vi "Quit LabVIEW.vi"(8 "error in (no error)":errorcluster) -> ()   [LabVIEW 2018]
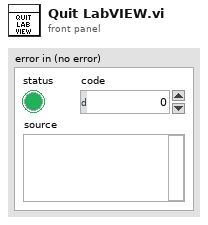
[diagram p1: front panel]
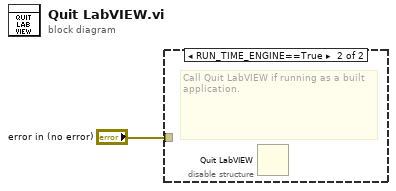
[diagram p0: block diagram]
diagram:
  n1 = disable-structure shown="RUN_TIME_ENGINE==True" {
    disable-tunnel: "error in (no error)" -> [_ _]
    frame condition #0 (active) {
    }
    frame condition #1 {
      # "Call Quit LabVIEW if running as a built application."
      n2 = Quit LabVIEW() -> ()  [unwired: 1 in]
    }
  }
